vi "Get All DMA Channels.vi"(8 "error in (no error)":errorcluster, 11 "FPGA addon refnum in":T1 format="%.0x") -> (0 "error out":errorcluster, 2 "DMA channels out":T2[](array[typedef]) {"Data Type" format="%.0x"}, 3 "FPGA addon refnum out":T1=18446744073709551615 format="%.0x")   [LabVIEW 2021, in "FPGA Addon Bitfile Reload Unit Tests.lvclass"]
uses:
  FPGA Addon Bitfile Reload Unit Tests.lvclass
  Addon/Addon Shared/Types/DMA Information.ctl
  Addon/Addon Shared/Types/FPGA Addon Data Type.ctl
  <vilib>/NI VeriStand/Custom Device API/Custom Device Item Ref.ctl
  Addon/Addon Shared/Types/FG Action.ctl
  Addon/Addon Shared/SubVIs/Constants.vi
  <vilib>/NI VeriStand/Custom Device Tools/Custom Device Utility Library/NI VeriStand - Search for Item by GUID.vi
  <vilib>/NI/NI VeriStand Advanced SysDef API/SysDef API/SysDef.Property.Get.vi
  <vilib>/NI/NI VeriStand Advanced SysDef API/_SubVIs/SysDef.Property.Get.Variant.vi
  <vilib>/NI/NI VeriStand Advanced SysDef API/SysDef API/SysDef.Property.Set.vi
  <vilib>/NI/NI VeriStand Advanced SysDef API/_SubVIs/SysDef.Property.Set.Variant.vi
  Addon/Addon Shared/FPGA Addon Shared.lvlib
  <vilib>/NI VeriStand/Custom Device Tools/Custom Device Utility Library/Custom Device Utility Library.lvlib
  <vilib>/NI VeriStand/Custom Device API/Custom Device API.lvlib
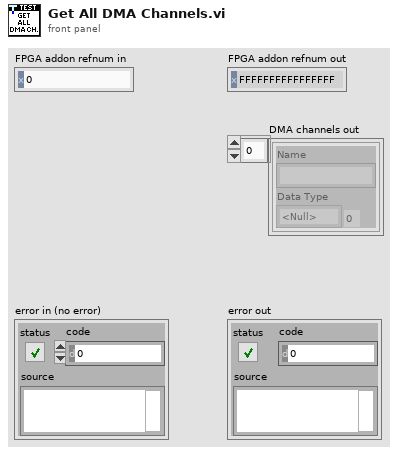
[diagram p1: front panel]
types:
  T1 = typedef "Custom Device API.lvlib/Custom Device Item Ref.ctl" = u64
  T2 = typedef "FPGA Addon Shared.lvlib/DMA Information.ctl" = cluster{"Name":string, "Data Type":T3}
  T3 = typedef "FPGA Addon Shared.lvlib/FPGA Addon Data Type.ctl" = enum8{"<Null>", "I8", "I16", "I32", "I64", "U8", "U16", "U32", "U64", "SGL", "Boolean", "Analog PWM In Settings", "Analog PWM In", "Digital PWM In Settings", "Digital PWM In", "Digital PWM Out", "Sine Out", "FXP", "FXP+/-24.5", "FXP+/-16.5", "FXP+/-32.8", "FXP+/-64.32", "FXP+/-16.7", "FXP+/-20.5", "FXP+/-27.5", "FXP+/-32.16", "FXP+16.3", "FXP+18.3", "Digital Static In", "Digital Static Out", "Digital Static In Settings", "Digital WSS Out", "Quad Encoder Settings", "Quad Encoder In", "Group"}
  T4 = typedef "FPGA Addon Shared.lvlib/FG Action.ctl" = enum8{"GET", "SET"}
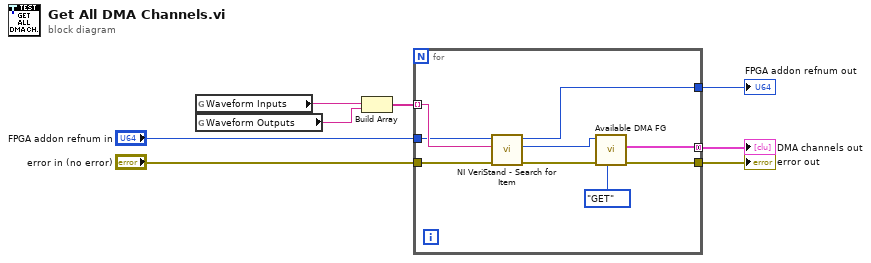
[diagram p0: block diagram]
diagram:
  n1 = global read "Constants.vi" "Waveform Inputs"() -> (w2:string)
  n2 = global read "Constants.vi" "Waveform Outputs"() -> (w3:string)
  n3 = Build Array(w2, w3) -> (w6:string[])
  n4 = for {
    tunnel: "error in (no error)" -> [w17]
    tunnel: "FPGA addon refnum in" -> [w14]
    tunnel: w6 -> [w15] mode=indexing
    tunnel: [w12] -> w8 mode=concatenating
    tunnel: [w11] -> w7
    tunnel: [w10] -> w1
    n5 = call-poly <vilib>:"NI VeriStand - Search for Item.vi"("error in"=w17, "Item GUID"=w15, "Section Ref in"=w14) -> ("error out"=w16:errorcluster, "Item Ref"=w9:T1, "Section Ref out"=w10:T1)  [unwired: 5 in, 1 out]
    n6 = call "Available DMA FG.vi"("Action"=FG_Action."GET", "error in (no error)"=w16, "Item Ref"=w9) -> ("error out"=w11:errorcluster, "Available DMA"=w12:T2[])  [unwired: 6 in, 1 out]
  }
  "DMA channels out" <- w8
  "error out" <- w7
  "FPGA addon refnum out" <- w1
